vi "hokuyo_closestObject.vi"(1 "Current stepper angle":dbl, 2 "Array":cluster{"Magnitude":dbl, "Direction":dbl}[](array[cluster])) -> (0 "Target Direction":dbl)   [LabVIEW 2014]
panel:
  out "Object Distance":dbl
  in  "stop":bool
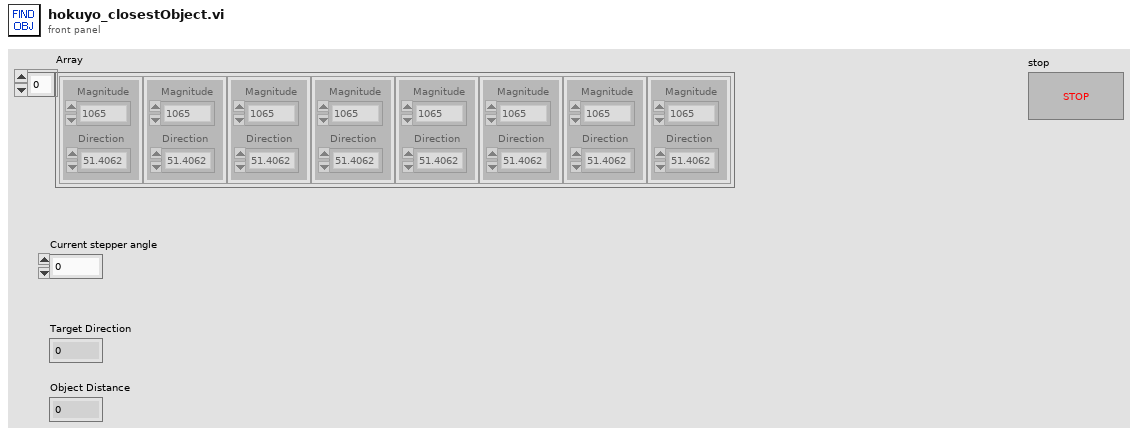
[diagram p1: front panel]
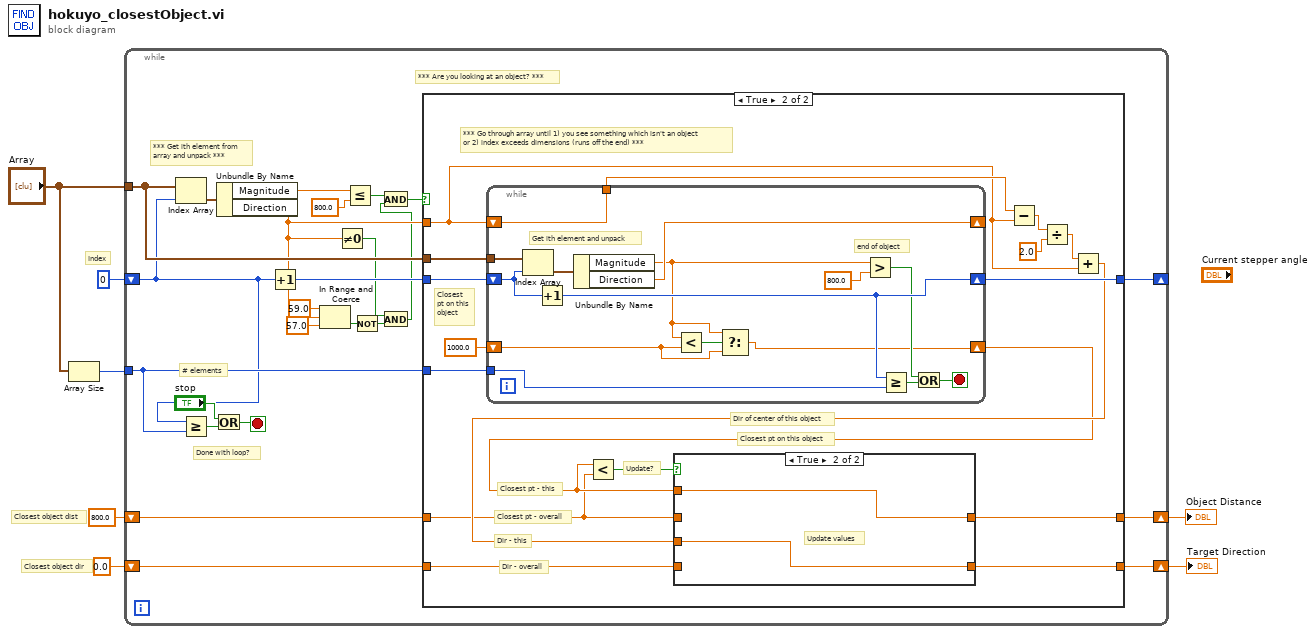
[diagram p0: block diagram]
diagram:
  # "Index"
  # "Closest object dir"
  # "Closest object dist"
  n1 = Array Size(array="Array") -> (size(s)=w2:i32)
  n2 = while {
    tunnel: "Array" -> [w30]
    shift-right: [w31] -> _
    shift-left: 0 -> [w19]
    shift-right: [w22] -> w4
    shift-left: 800.0 -> [w28]
    shift-right: [w21] -> w3
    shift-left: 0.0 ("Largest Hole Direction") -> [w29]
    tunnel: w2 -> [w23]
    stop <- w27 stop-if-true
    # "# elements"
    # "Done with loop?"
    # "*** Are you looking at an object? ***"
    # "*** Get ith element from \narray and unpack ***"
    n3 = Index Array(array=w30, index=w19) -> (element=w18:cluster{"Magnitude":dbl, "Direction":dbl})
    n4 = Greater Or Equal?(x=w19, y=w23) -> (x >= y?=w26:bool)
    n5 = Or(x="stop", y=w26) -> (x .or. y?=w27:bool)
    n6 = Unbundle By Name(w18) -> ("Magnitude"=w16:dbl, "Direction"=w14:dbl)
    n7 = Increment(x=w19) -> (x+1=w20:i32)
    n8 = In Range and Coerce(upper limit=59.0, x=w14, lower limit=57.0) -> (In Range?=w11:bool)  [unwired: 1 out]
    n9 = Not Equal To 0?(x=w14) -> (x != 0?=w10:bool)
    n10 = Less Or Equal?(x=w16, y=800.0) -> (x <= y?=w15:bool)
    n11 = Not(x=w11) -> (.not. x?=w8:bool)
    n12 = And(x=w10, y=w8) -> (x .and. y?=w9:bool)
    n13 = And(x=w15, y=w9) -> (x .and. y?=w17:bool)
    n14 = case shown="True" w17 {
      tunnel: w20 -> [w34 w51]
      tunnel: [w34 w45] -> w31
      tunnel: w30 -> [_ w50]
      tunnel: w14 -> [_ w35]
      tunnel: w29 -> [w33 w41]
      tunnel: w28 -> [w32 w37]
      tunnel: [w33 w47] -> w21
      tunnel: [w32 w39] -> w22
      tunnel: w23 -> [_ w44]
      frame False {
        # "*** Keep looking for the beginning of a hole ***"
      }
      frame True {
        # "Update?"
        # "Dir - overall"
        # "Dir - this"
        # "Closest pt - overall"
        # "Closest pt - this"
        # "Closest pt on this object"
        # "Closest\npt on this\nobject"
        # "Dir of center of this object"
        # "*** Go through array until 1) you see something which isn't an object \nor 2) index exceeds dimensions (runs off the end) ***"
        n15 = while {
          tunnel: w50 -> [w70]
          shift-right: [w65] -> w45
          shift-left: w51 -> [w67]
          tunnel: w44 -> [w64]
          shift-right: [w62] -> _
          shift-left: w35 -> [w61]
          tunnel: [w61] -> w43
          shift-right: [w56] -> w38
          shift-left: 1000.0 -> [w58]
          stop <- w66 stop-if-true
          # "end of object"
          # "Get ith element and unpack"
          n16 = Index Array(array=w70, index=w67) -> (element=w68:cluster{"Magnitude":dbl, "Direction":dbl})
          n17 = Increment(x=w67) -> (x+1=w65:i32)
          n18 = Unbundle By Name(w68) -> ("Magnitude"=w57:dbl, "Direction"=w62:dbl)
          n19 = Less?(x=w57, y=w58) -> (x < y?=w59:bool)
          n20 = Select(t=w57, s=w59, f=w58) -> (s? t:f=w56:dbl)
          n21 = Greater?(x=w57, y=800.0) -> (0:w60:bool)
          n22 = Greater Or Equal?(x=w65, y=w64) -> (x >= y?=w63:bool)
          n23 = Or(x=w60, y=w63) -> (x .or. y?=w66:bool)
        }
        n24 = Less?(x=w38, y=w37) -> (x < y?=w36:bool)
        n25 = Subtract(x=w43, y=w35) -> (x-y=w46:dbl)
        n26 = Divide(x=w46, y=2.0) -> (x/y=w48:dbl)
        n27 = Add(x=w48, y=w35) -> (x+y=w42:dbl)
        n28 = case shown="True" w36 {
          tunnel: w42 -> [_ w55]
          tunnel: w41 -> [w53 _]
          tunnel: [w53 w55] -> w47
          tunnel: w38 -> [_ w54]
          tunnel: w37 -> [w52 _]
          tunnel: [w52 w54] -> w39
          frame False {
            # "Keep old values"
          }
          frame True {
            # "Update values"
          }
        }
      }
    }
  }
  "Object Distance" <- w4
  "Target Direction" <- w3
